vi "Abort API.vi"(8 "error in (no error)":errorcluster, 11 "TopLevel in":refnum<class "TopLevel.lvclass">) -> (0 "error out":errorcluster, 3 "TopLevel out":refnum<class "TopLevel.lvclass">)   [LabVIEW 2022 SP3, in "TopLevel.lvclass"]
uses:
  TopLevel.lvclass
  Typedefs/API Command Cluster.ctl
  Typedefs/API Command Enum.ctl
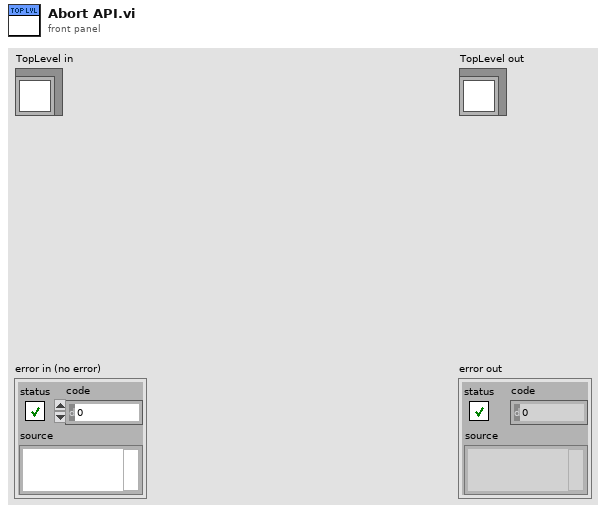
[diagram p1: front panel]
types:
  T1 = typedef "TopLevel.lvclass/API Command Enum.ctl" = enum16{"Execute Printer Commands", "Pre Purge", "Enable Ink Ch-1", "Enable Ink Ch-2", "Enable Ink Ch-3", "Enable Ink Ch-4", "Enable Ink Ch-5", "Enable Ink Ch-6", "Disable Ink Ch-1", "Disable Ink Ch-2", "Disable Ink Ch-3", "Disable Ink Ch-4", "Disable Ink Ch-5", "Disable Ink Ch-6", "ExecuteIdlePrintCycle", "StopIdlePrintCycle", "Abort", "LoadDLP2GUIConfig", "SaveDLP2GUIConfig", "PrimingMode", "SetHeadTemperature", "EnableHead", "EnableHeadHeat", "SetSystemMode", "HeadPrint", "AbortAll", "Send Printer String"}
  T2 = typedef "TopLevel.lvclass/API Command Cluster.ctl" = cluster{"Command":T1, "Arguments":string, "Data":variant}
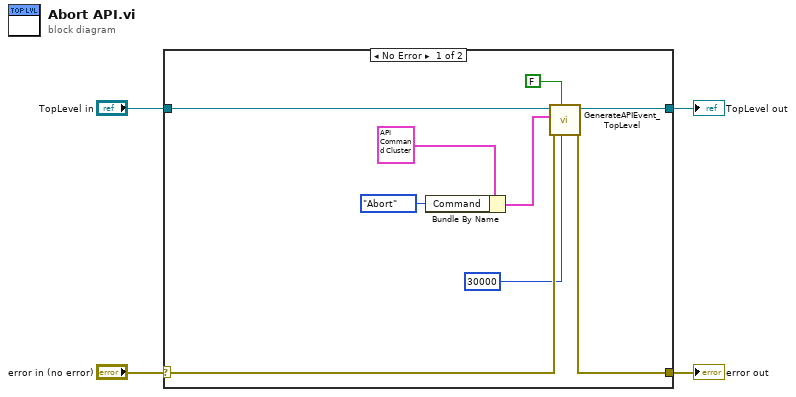
[diagram p0: block diagram]
diagram:
  n1 = case shown="No Error" "error in (no error)" {
    selector: "error in (no error)" -> [w11 w15]
    tunnel: [w10 w15] -> w3
    tunnel: [w13 w14] -> w1
    tunnel: "TopLevel in" -> [w12 w14]
    frame No Error {
      n2 = Bundle By Name(cluster=T2 {"Command"=enum."Execute Printer Commands", "Arguments"="", "Data"=variant} ("API Command Cluster"), "Command"=API_Command_Enum."Abort") -> (w7:T2)
      n3 = call-dynamic "GenerateAPIEvent_TopLevel.vi"("Timeout (ms)"=u32 30000, "Wait (F)"=FALSE, "error in (no error)"=w11, "API Command Cluster"=w7, "TopLevel in"=w12) -> ("error out"=w10:errorcluster, "TopLevel out"=w13:refnum<class "TopLevel.lvclass">)  [unwired: 5 in]
    }
    frame Error {
    }
  }
  "error out" <- w3
  "TopLevel out" <- w1
